vi "sub_webcam.vi"(5 "Session In":T2) -> (0 "Video Image":T1(plugin-control), 1 "error out":errorcluster, 2 "Data String":string)   [LabVIEW 2014]
uses:
  <vilib>/userdefined/High Color/IMAQdx.ctl
  <vilib>/vision/driver/NI_Vision_Acquisition_Software.lvlib
panel:
  out "Image Pixels array":u32[][](array[numeric])
  in  "stop":bool
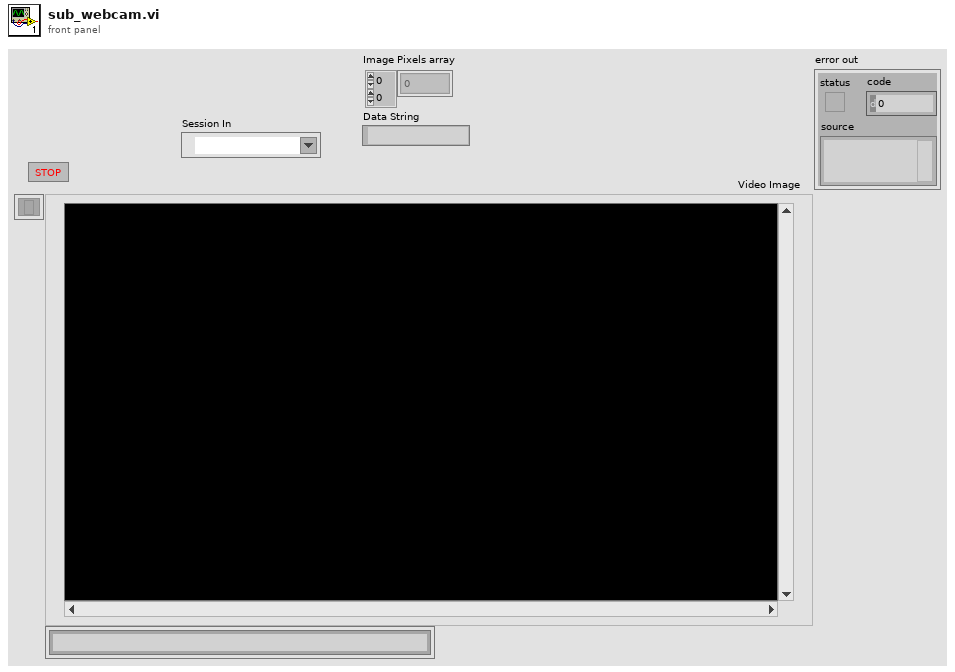
[diagram p1: front panel]
types:
  T1 = typedef "IMAQ Image.ctl" = refnum<image>
  T2 = typedef "IMAQdx.ctl" = refnum<k21>
  T3 = typedef "Image Type" = u32
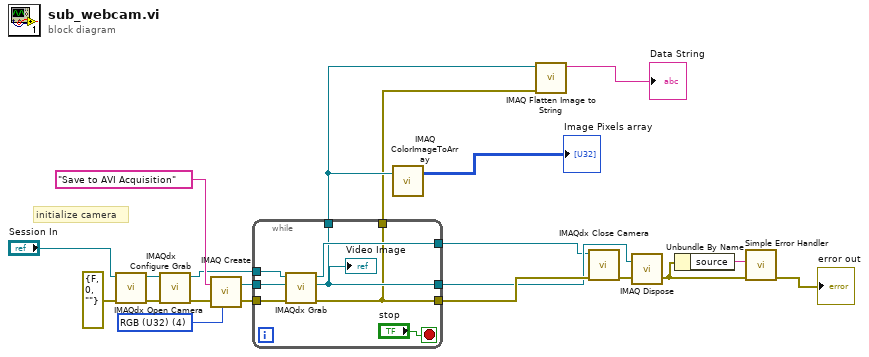
[diagram p0: block diagram]
diagram:
  w21 = T3 4 items=["Grayscale (U8)", "Grayscale (I16)", "Grayscale (SGL)", "Complex (CSG)", "RGB (U32)", "HSL (U32)", "RGB (U64)", "Grayscale (U16)"] ("Image Type")
  # "initialize camera"
  n1 = call <vilib>:"IMAQdx Open Camera.vi"("error in"=errorcluster {"status"=FALSE, "code"=0, "source"=""}, "Session In"="Session In") -> ("error out"=w8:errorcluster, "Session Out"=w19:T2)  [unwired: 8 in]
  n2 = call <vilib>:"IMAQdx Configure Grab.vi"("error in"=w8, "Session In"=w19) -> ("error out"=w7:errorcluster, "Session Out"=w16:T2)  [unwired: 8 in]
  n3 = call "IMAQ Create"("Image Name"="Save to AVI Acquisition", "Image Type"=w21, "error in (no error)"=w7) -> ("New Image"=w11:T1, "error out"=w6:errorcluster)  [unwired: 2 in]
  n4 = while {
    tunnel: w16 -> [w28]
    tunnel: [w22] -> w13
    tunnel: [w23] -> w12
    tunnel: w11 -> [w27]
    tunnel: [w26] -> w10
    tunnel: w6 -> [w24]
    tunnel: [w23] -> w4
    tunnel: [w22] -> w2
    stop <- "stop" stop-if-true
    n5 = call <vilib>:"IMAQdx Grab.vi"("error in"=w24, "Image In"=w27, "Session In"=w28) -> ("error out"=w22:errorcluster, "Image Out"=w23:T1, "Session Out"=w26:T2)  [unwired: 5 in, 1 out]
    "Video Image" <- w23
  }
  n6 = call "IMAQ ColorImageToArray"("Image"=w4) -> ("Image Pixels (U32)"=→"Image Pixels array":u32[][])  [unwired: 3 in, 2 out]
  n7 = call "IMAQ Flatten Image to String"("error in (no error)"=w2, "Image"=w4) -> ("Data String"=→"Data String":string)  [unwired: 8 in, 1 out]
  n8 = call <vilib>:"IMAQdx Close Camera.vi"("error in"=w13, "Session In"=w10) -> ("error out"=w9:errorcluster)  [unwired: 9 in]
  n9 = call "IMAQ Dispose"("Image"=w12, "error in (no error)"=w9) -> ("error out"=w15:errorcluster)  [unwired: 1 in, 3 out]
  n10 = Unbundle By Name(w15) -> ("source"=w14:string)
  n11 = call <vilib>:"Simple Error Handler.vi"("error source (\" \")"=w14, "error in (no error)"=w15) -> ("error out"=→"error out":errorcluster)  [unwired: 3 in, 4 out]
